vi "Convert Table to VI Information Array.vi"(11 "Array Out":string[][](array[string])) -> (3 "VI Information Array":T1[](array[typedef]))   [LabVIEW 2017, in "Engine.lvclass"]
uses:
  Engine.lvclass
  VI Information.ctl
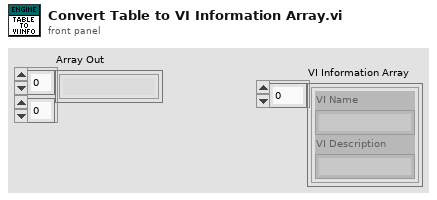
[diagram p1: front panel]
types:
  T1 = typedef "Engine.lvclass/VI Information.ctl" = cluster{"VI Name":string, "VI Description":string}
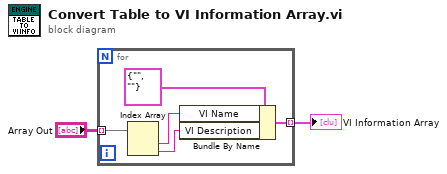
[diagram p0: block diagram]
diagram:
  n1 = for {
    tunnel: "Array Out" -> [w5] mode=indexing
    tunnel: [w6] -> w1 mode=indexing
    n2 = Index Array(array=w5) -> (element #1=w4:string, element #2=w3:string)  [unwired: 2 in]
    n3 = Bundle By Name(cluster=T1 {"VI Name"="", "VI Description"=""} ("VI Information"), "VI Name"=w4, "VI Description"=w3) -> (w6:T1)
  }
  "VI Information Array" <- w1
